vi "Read Loop Async.vi"(11 "Terminal in":refnum<class "Terminal.lvclass">) -> ()   [LabVIEW 2020, in "Terminal.lvlib" / "Terminal.lvclass"]
uses:
  Terminal.lvclass
  Terminal.lvclass/Terminal.ctl
  <vilib>/IlluminatedG/lv-stream/Connection/Connection.lvclass
  <vilib>/IlluminatedG/lv-stream/stream/Stream.lvclass
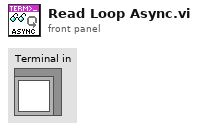
[diagram p1: front panel]
types:
  T1 = typedef "Terminal.lvlib/Terminal.lvclass/Ref Data.ctl" = cluster{"Connection":refnum<class "Connection.lvclass">, "Read Loop Running":bool, "Parse State":T2, "Terminal Options":T7, "Font Metrics":T10, "Scroll":i32, "Close Read Loop":bool, "Buffer":T11, "Pause Read Loop":bool}
  T2 = typedef "Terminal.lvlib/Terminal.lvclass/Parse State.ctl" = cluster{"Buffer State":T3, "Cursor":T4, "Attributes":T6}
  T3 = typedef "Terminal.lvlib/Terminal.lvclass/Buffer State.ctl" = cluster{"Sequence":string, "ESC":bool, "Alt Buf":bool}
  T4 = typedef "Terminal.lvlib/Terminal.lvclass/Cursor.ctl" = cluster{"Cur":T5, "Saved":T5}
  T5 = typedef "Terminal.lvlib/Terminal.lvclass/Position.ctl" = cluster{"Row":i32, "Col":i32}
  T6 = typedef "Terminal.lvlib/Text Attributes.ctl" = cluster{"FG":u32, "BG":u32, "Bold":bool, "Italic":bool, "Underline":bool, "Strike":bool, "Inverse":bool}
  T7 = typedef "Terminal.lvlib/Terminal Options.ctl" = cluster{"Implied CR with LF":bool, "Local Echo":bool, "Tab Width":i32, "Color Scheme":T8, "Default FG":T9, "Default BG":T9, "History Length":i32, "Font Face":string, "Font Size":i16, "Rows":i32, "Cols":i32}
  T8 = typedef "Terminal.lvlib/Color Scheme.ctl" = cluster{"Black":u32, "Red":u32, "Green":u32, "Yellow":u32, "Blue":u32, "Magenta":u32, "Cyan":u32, "White":u32, "Bright Black":u32, "Bright Red":u32, "Bright Green":u32, "Bright Yellow":u32, "Bright Blue":u32, "Bright Magenta":u32, "Bright Cyan":u32, "Bright White":u32}
  T9 = typedef "Terminal.lvlib/Color.ctl" = i8
  T10 = typedef "Terminal.lvlib/Terminal.lvclass/Font Metrics.ctl" = cluster{"Width":i16, "Height":i16}
  T11 = typedef "Terminal.lvlib/Buffer.ctl" = enum16{"Primary", "Alternate"}
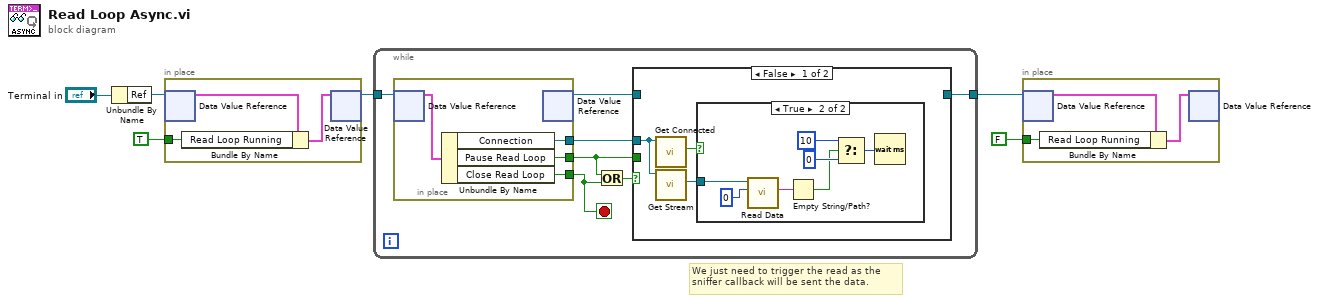
[diagram p0: block diagram]
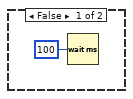
[diagram p2: hidden frame]
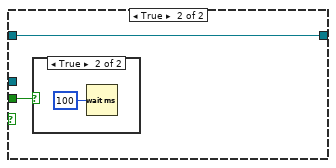
[diagram p3: hidden frame]
diagram:
  # "We just need to trigger the read as the sniffer callback will be sent the data."
  n1 = Unbundle By Name("Terminal in") -> ("Ref"=w5:refnum<data-value>)
  n2 = in-place {
    in-place-border: TRUE ("Read Loop Running") -> [w8]
    n3 = in-place-dvr #1(w5) -> (w9:T1)  [unwired: 1 out]
    n4 = Bundle By Name(cluster=w9, "Read Loop Running"=w8) -> (w7:T1)
    n5 = in-place-dvr #1(w7) -> (w3:refnum<data-value>)  [unwired: 1 out]
  }
  n6 = while {
    tunnel: w3 -> [w15]
    tunnel: [w13] -> w1
    stop <- w12 stop-if-true
    n7 = in-place {
      in-place-border: [w19] -> w16
      in-place-border: [w18] -> w12
      in-place-border: [w17] -> w10
      n8 = in-place-dvr #2(w15) -> (w20:T1)  [unwired: 1 out]
      n9 = Unbundle By Name(w20) -> ("Connection"=w19:refnum<class "Connection.lvclass">, "Pause Read Loop"=w17:bool, "Close Read Loop"=w18:bool)
      n10 = in-place-dvr #2() -> (w14:refnum<data-value>)  [unwired: 1 in, 1 out]
    }
    n11 = Or(x=w10, y=w12) -> (x .or. y?=w11:bool)
    n12 = case shown="False" w11 {
      tunnel: w16 -> [w22 _]
      tunnel: w14 -> [_ w33]
      tunnel: [_ w33] -> w13
      tunnel: w10 -> [_ w32]
      frame False {
        n13 = call <vilib>:"Get Connected.vi"("Connection in"=w22) -> ("Connected"=w23:bool)  [unwired: 8 in, 2 out]
        n14 = call-dynamic "Get Stream.vi"("Connection in"=w22) -> ("Stream"=w21:refnum<class "Stream.lvclass">)  [unwired: 8 in, 2 out]
        n15 = case shown="True" w23 {
          tunnel: w21 -> [_ w31]
          frame False {
            n16 = Wait (ms)(milliseconds to wait=u32 100) -> ()  [unwired: 1 out]
          }
          frame True {
            n17 = call <vilib>:"Read Data.vi"("Count"=0, "Stream in"=w31) -> ("Data"=w29:string)  [unwired: 7 in, 2 out]
            n18 = Empty String/Path?(string/path=w29) -> (empty?=w25:bool)
            n19 = Select(t=u32 10 ("milliseconds to wait"), s=w25, f=u32 0 ("milliseconds to wait")) -> (s? t:f=w26:u32)
            n20 = Wait (ms)(milliseconds to wait=w26) -> ()  [unwired: 1 out]
          }
        }
      }
      frame True {
        n21 = case shown="True" w32 {
          frame False {
          }
          frame True {
            n22 = Wait (ms)(milliseconds to wait=u32 100) -> ()  [unwired: 1 out]
          }
        }
      }
    }
  }
  n23 = in-place {
    in-place-border: FALSE ("Read Loop Running") -> [w36]
    n24 = in-place-dvr #3(w1) -> (w37:T1)  [unwired: 1 out]
    n25 = Bundle By Name(cluster=w37, "Read Loop Running"=w36) -> (w35:T1)
    n26 = in-place-dvr #3(w35) -> ()  [unwired: 2 out]
  }
